vi "Analysis.Determine.vi"(8 "error in (no error)":errorcluster, 10 "Results":variant, 11 "Data Path":path) -> (0 "error out":errorcluster, 1 "Passed?":bool, 3 "Data Path":path)   [LabVIEW 2015, in "Analysis.lvlib"]
uses:
  Analysis.lvlib
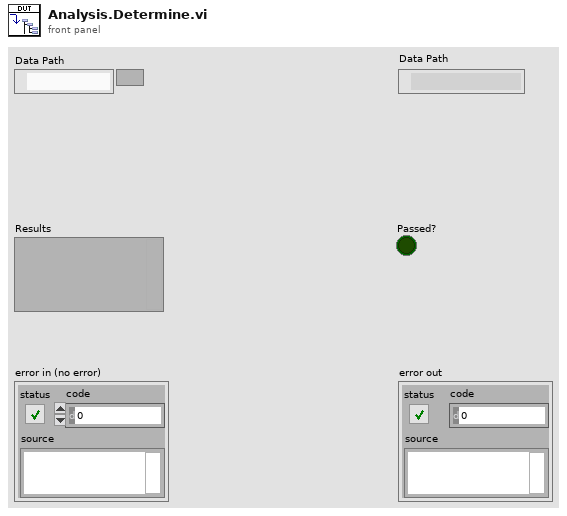
[diagram p1: front panel]
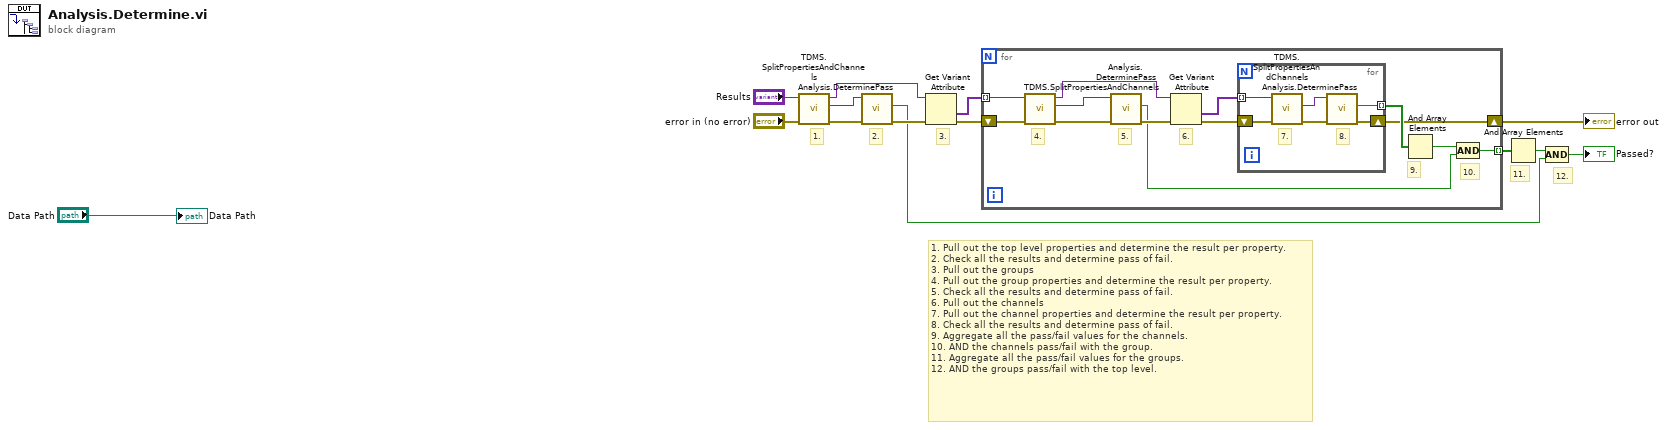
[diagram p0: block diagram]
diagram:
  # "1. Pull out the top level properties and determine the result per property.\n2. Check all the results and determine pass of fail.\n3. Pull out the groups\n4. Pull out the group properties and determine the result per property.\n5. Check all the results and determine pass of fail.\n6. Pull out the channels\n7. Pull out the channel properties and determine the result per property.\n8. Check all the results and determine pass of fail.\n9. Aggregate all the pass/fail values for the channels.\n10. AND the channels pass/fail with the group.\n11. Aggregate all the pass/fail values for the groups.\n12. AND the groups pass/fail with the top level."
  # "12."
  # "11."
  # "3."
  # "2."
  # "1."
  n1 = call "TDMS.SplitPropertiesAndChannels.vi"("error in"="error in (no error)", "Properties"="Results") -> ("error out"=w5:errorcluster, "Properties"=w1:variant, "Channels"=w12:variant)  [unwired: 7 in]
  n2 = call "Analysis.DeterminePass.vi"("error in (no error)"=w5, "Properties"=w1) -> ("error out"=w11:errorcluster, "Passed?"=w6:bool)  [unwired: 8 in]
  n3 = Get Variant Attribute(Variant=w12, error in=w11) -> (values=w9:variant[], error out=w10:errorcluster)  [unwired: 2 in, 2 out]
  n4 = for {
    tunnel: w9 -> [w23] mode=indexing
    shift-right: [w16] -> w2
    shift-left: w10 -> [w15]
    tunnel: [w17] -> w14 mode=indexing
    # "10."
    # "9."
    # "6."
    # "5."
    # "4."
    n5 = call "TDMS.SplitPropertiesAndChannels.vi"("error in"=w15, "Properties"=w23) -> ("error out"=w21:errorcluster, "Properties"=w19:variant, "Channels"=w22:variant)  [unwired: 7 in]
    n6 = call "Analysis.DeterminePass.vi"("error in (no error)"=w21, "Properties"=w19) -> ("error out"=w20:errorcluster, "Passed?"=w18:bool)  [unwired: 8 in]
    n7 = Get Variant Attribute(Variant=w22, error in=w20) -> (values=w25:variant[], error out=w26:errorcluster)  [unwired: 2 in, 2 out]
    n8 = for {
      shift-right: [w28] -> w16
      shift-left: w26 -> [w33]
      tunnel: w25 -> [w31] mode=indexing
      tunnel: [w32] -> w24 mode=indexing
      # "8."
      # "7."
      n9 = call "TDMS.SplitPropertiesAndChannels.vi"("error in"=w33, "Properties"=w31) -> ("error out"=w30:errorcluster, "Properties"=w29:variant)  [unwired: 7 in, 1 out]
      n10 = call "Analysis.DeterminePass.vi"("error in (no error)"=w30, "Properties"=w29) -> ("error out"=w28:errorcluster, "Passed?"=w32:bool)  [unwired: 8 in]
    }
    n11 = And Array Elements(Boolean array=w24) -> (logical AND=w27:bool)
    n12 = Compound Arithmetic op=AND(w27, w18) -> (w17:bool)
  }
  "error out" <- w2
  n13 = And Array Elements(Boolean array=w14) -> (logical AND=w8:bool)
  n14 = Compound Arithmetic op=AND(w8, w6) -> (→"Passed?":bool)
  "Data Path" <- "Data Path"
